vi "ArmUnitsToInches.vi"(11 "Sensor Units":i32) -> (2 "Angle":dbl, 3 "Inches":dbl)   [LabVIEW 2018]
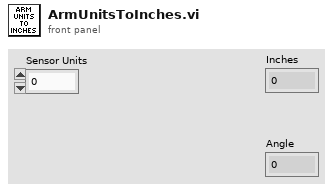
[diagram p1: front panel]
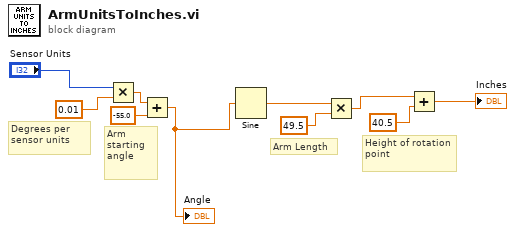
[diagram p0: block diagram]
diagram:
  # "Arm starting angle"
  # "Degrees per sensor units"
  # "Height of rotation point"
  # "Arm Length"
  n1 = Multiply(x="Sensor Units", y=0.01) -> (x*y=w8:dbl)
  n2 = Add(x=w8, y=-55.0) -> (x+y=w6:dbl)
  "Angle" <- w6
  n3 = Sine(x=w6) -> (sin(x)=w5:dbl)
  n4 = Multiply(x=w5, y=49.5) -> (x*y=w3:dbl)
  n5 = Add(x=w3, y=40.5) -> (x+y=→"Inches":dbl)
